vi "Begin.vi"(8 "error in":errorcluster) -> (0 "error out":errorcluster)   [LabVIEW 2020]
doc: "Called before other user functions, this VI is expected to open initial I/O refnums, load in file data, and do all program initialization. Notice that the <B>error out</B> terminal is simply used for data flow. Wiring it to other structures or subVIs ensures that this VI runs first."
uses:
  <vilib>/Rock Robotics/WPI/ThirdParty/Phoenix-LabVIEW/CANCoder/Controls/CTRE_Phoenix_CANcoder_Configurables.ctl
  <vilib>/Rock Robotics/WPI/ThirdParty/Phoenix-LabVIEW/CANCoder/Controls/CTRE_Phoenix_CANcoder_SensorInitializationStrategy.ctl
  <vilib>/Rock Robotics/WPI/ThirdParty/Phoenix-LabVIEW/CANCoder/Controls/CTRE_Phoenix_CANcoder_AbsoluteSensorRange.ctl
  <vilib>/Rock Robotics/WPI/ThirdParty/Phoenix-LabVIEW/Motor Controller/Controls/CTRE_Phoenix_MotorControl_VelocityMeasurementPeriod.ctl
  <vilib>/Rock Robotics/WPI/ThirdParty/Phoenix-LabVIEW/CANCoder/Controls/CTRE_Phoenix_CANcoder_SensorTimeBase.ctl
  <vilib>/Rock Robotics/WPI/DriverStation/WPI_DriverStationRobotMode2.ctl
  <vilib>/Rock Robotics/WPI/Joystick/WPI_JoystickDeviceEnum.ctl
  <vilib>/Rock Robotics/WPI/ThirdParty/Phoenix-LabVIEW/Pigeon IMU/CTRE_PigeonIMU_TareType.ctl
  <vilib>/Rock Robotics/WPI/ThirdParty/Phoenix-LabVIEW/Motor Controller/Controls/CTRE_Phoenix_MotorControl_TalonFXInvertType.ctl
  <vilib>/Rock Robotics/WPI/ThirdParty/Phoenix-LabVIEW/Motor Controller/Controls/CTRE_Phoenix_MotorControl_NeutralMode.ctl
  <vilib>/Rock Robotics/WPI/ThirdParty/Phoenix-LabVIEW/Motor Controller/Controls/CTRE_Phoenix_MotorControl_SupplyCurrentLimitConfiguration.ctl
  <vilib>/Rock Robotics/WPI/ThirdParty/Phoenix-LabVIEW/Motor Controller/Controls/CTRE_Phoenix_MotorControl_FeedbackDevice_TalonFX.ctl
  <vilib>/Rock Robotics/WPI/ThirdParty/REV Robotics/REVLib/Typedef/Spark MAX Idle Mode.ctl
  <vilib>/Rock Robotics/WPI/ThirdParty/REV Robotics/REVLib/Typedef/Spark MAX Limit Direction.ctl
  <vilib>/Rock Robotics/WPI/ThirdParty/Phoenix-LabVIEW/Motor Controller/Controls/CTRE_Phoenix_MotorControl_FeedbackDevice.ctl
  <vilib>/Rock Robotics/SystemInterfaces/DIO/FPGA_DIOChannel.ctl
  <vilib>/Rock Robotics/SystemInterfaces/AnalogTrigger/FPGA_AnalogTriggerOutType.ctl
  <vilib>/Rock Robotics/SystemInterfaces/DIO/FPGA_DIOPWMChannel.ctl
  <vilib>/Rock Robotics/WPI/ThirdParty/JAS_Junk/TrajLib/Rotation2d_CreateAngle.vi
  <vilib>/Rock Robotics/WPI/ThirdParty/JAS_Junk/TrajLib/Translation2d_Create.vi
  Robot Global Data.vi
  <vilib>/Rock Robotics/WPI/ThirdParty/Phoenix-LabVIEW/CANCoder/Set/CTRE_Phoenix_CANcoder_SetPositionToAbsolute.vi
  <vilib>/Rock Robotics/WPI/Counter/WPI_CounterDigitalInputToDigitalSource.vi
  <vilib>/Rock Robotics/WPI/AnalogTrigger/WPI_AnalogTriggerOpen_DutyCycle.vi
  <vilib>/Rock Robotics/WPI/Counter/WPI_CounterAnalogTriggerToDigitalSource.vi
  <vilib>/Rock Robotics/WPI/Counter/WPI_CounterOpen UpDown Mode.vi
  <vilib>/Rock Robotics/WPI/MotorControl/WPI_MotorControlOpen SPARK.vi
  <vilib>/Rock Robotics/WPI/ThirdParty/JAS_Junk/TrajLib/Trajectory_Library.lvlib
panel:
  in  "CANcoder ID1":T1={"Sensor Initialization Strategy"=enum."Boot To Absolute Position", "Absolute Sensor Range"=enum."Signed [-180 to +180)", "Velocity Measurement Period"=100, "Velocity Measurement Window"=64, "Magnet Offset (Degrees)"=85.0, "Sensor Direction"=FALSE, "Sensor Coefficient"=0.087890625, "Unit String"="deg", "Sensor Time Base"=enum."PerMinute"} {"Velocity Measurement Period" items=["Period_1ms"=1, "Period_2ms"=2, "Period_5ms"=5, "Period_10ms"=10, "Period_20ms"=20, "Period_25ms"=25, "Period_50ms"=50, "Period_100ms"=100]; "Sensor Coefficient" format="%#_9g"}
  in  "CANcoder ID0":T1={"Sensor Initialization Strategy"=enum."Boot To Absolute Position", "Absolute Sensor Range"=enum."Signed [-180 to +180)", "Velocity Measurement Period"=100, "Velocity Measurement Window"=64, "Magnet Offset (Degrees)"=116.0, "Sensor Direction"=FALSE, "Sensor Coefficient"=0.087890625, "Unit String"="deg", "Sensor Time Base"=enum."PerMinute"} {"Velocity Measurement Period" items=["Period_1ms"=1, "Period_2ms"=2, "Period_5ms"=5, "Period_10ms"=10, "Period_20ms"=20, "Period_25ms"=25, "Period_50ms"=50, "Period_100ms"=100]; "Sensor Coefficient" format="%#_9g"}
  in  "CANcoder ID2":T1={"Sensor Initialization Strategy"=enum."Boot To Absolute Position", "Absolute Sensor Range"=enum."Signed [-180 to +180)", "Velocity Measurement Period"=100, "Velocity Measurement Window"=64, "Magnet Offset (Degrees)"=-75.0, "Sensor Direction"=FALSE, "Sensor Coefficient"=0.087890625, "Unit String"="deg", "Sensor Time Base"=enum."PerMinute"} {"Velocity Measurement Period" items=["Period_1ms"=1, "Period_2ms"=2, "Period_5ms"=5, "Period_10ms"=10, "Period_20ms"=20, "Period_25ms"=25, "Period_50ms"=50, "Period_100ms"=100]; "Sensor Coefficient" format="%#_9g"}
  in  "CANcoder ID3":T1={"Sensor Initialization Strategy"=enum."Boot To Absolute Position", "Absolute Sensor Range"=enum."Signed [-180 to +180)", "Velocity Measurement Period"=100, "Velocity Measurement Window"=-116, "Magnet Offset (Degrees)"=-134.0, "Sensor Direction"=FALSE, "Sensor Coefficient"=0.087890625, "Unit String"="deg", "Sensor Time Base"=enum."PerMinute"} {"Velocity Measurement Period" items=["Period_1ms"=1, "Period_2ms"=2, "Period_5ms"=5, "Period_10ms"=10, "Period_20ms"=20, "Period_25ms"=25, "Period_50ms"=50, "Period_100ms"=100]; "Sensor Coefficient" format="%#_9g"}
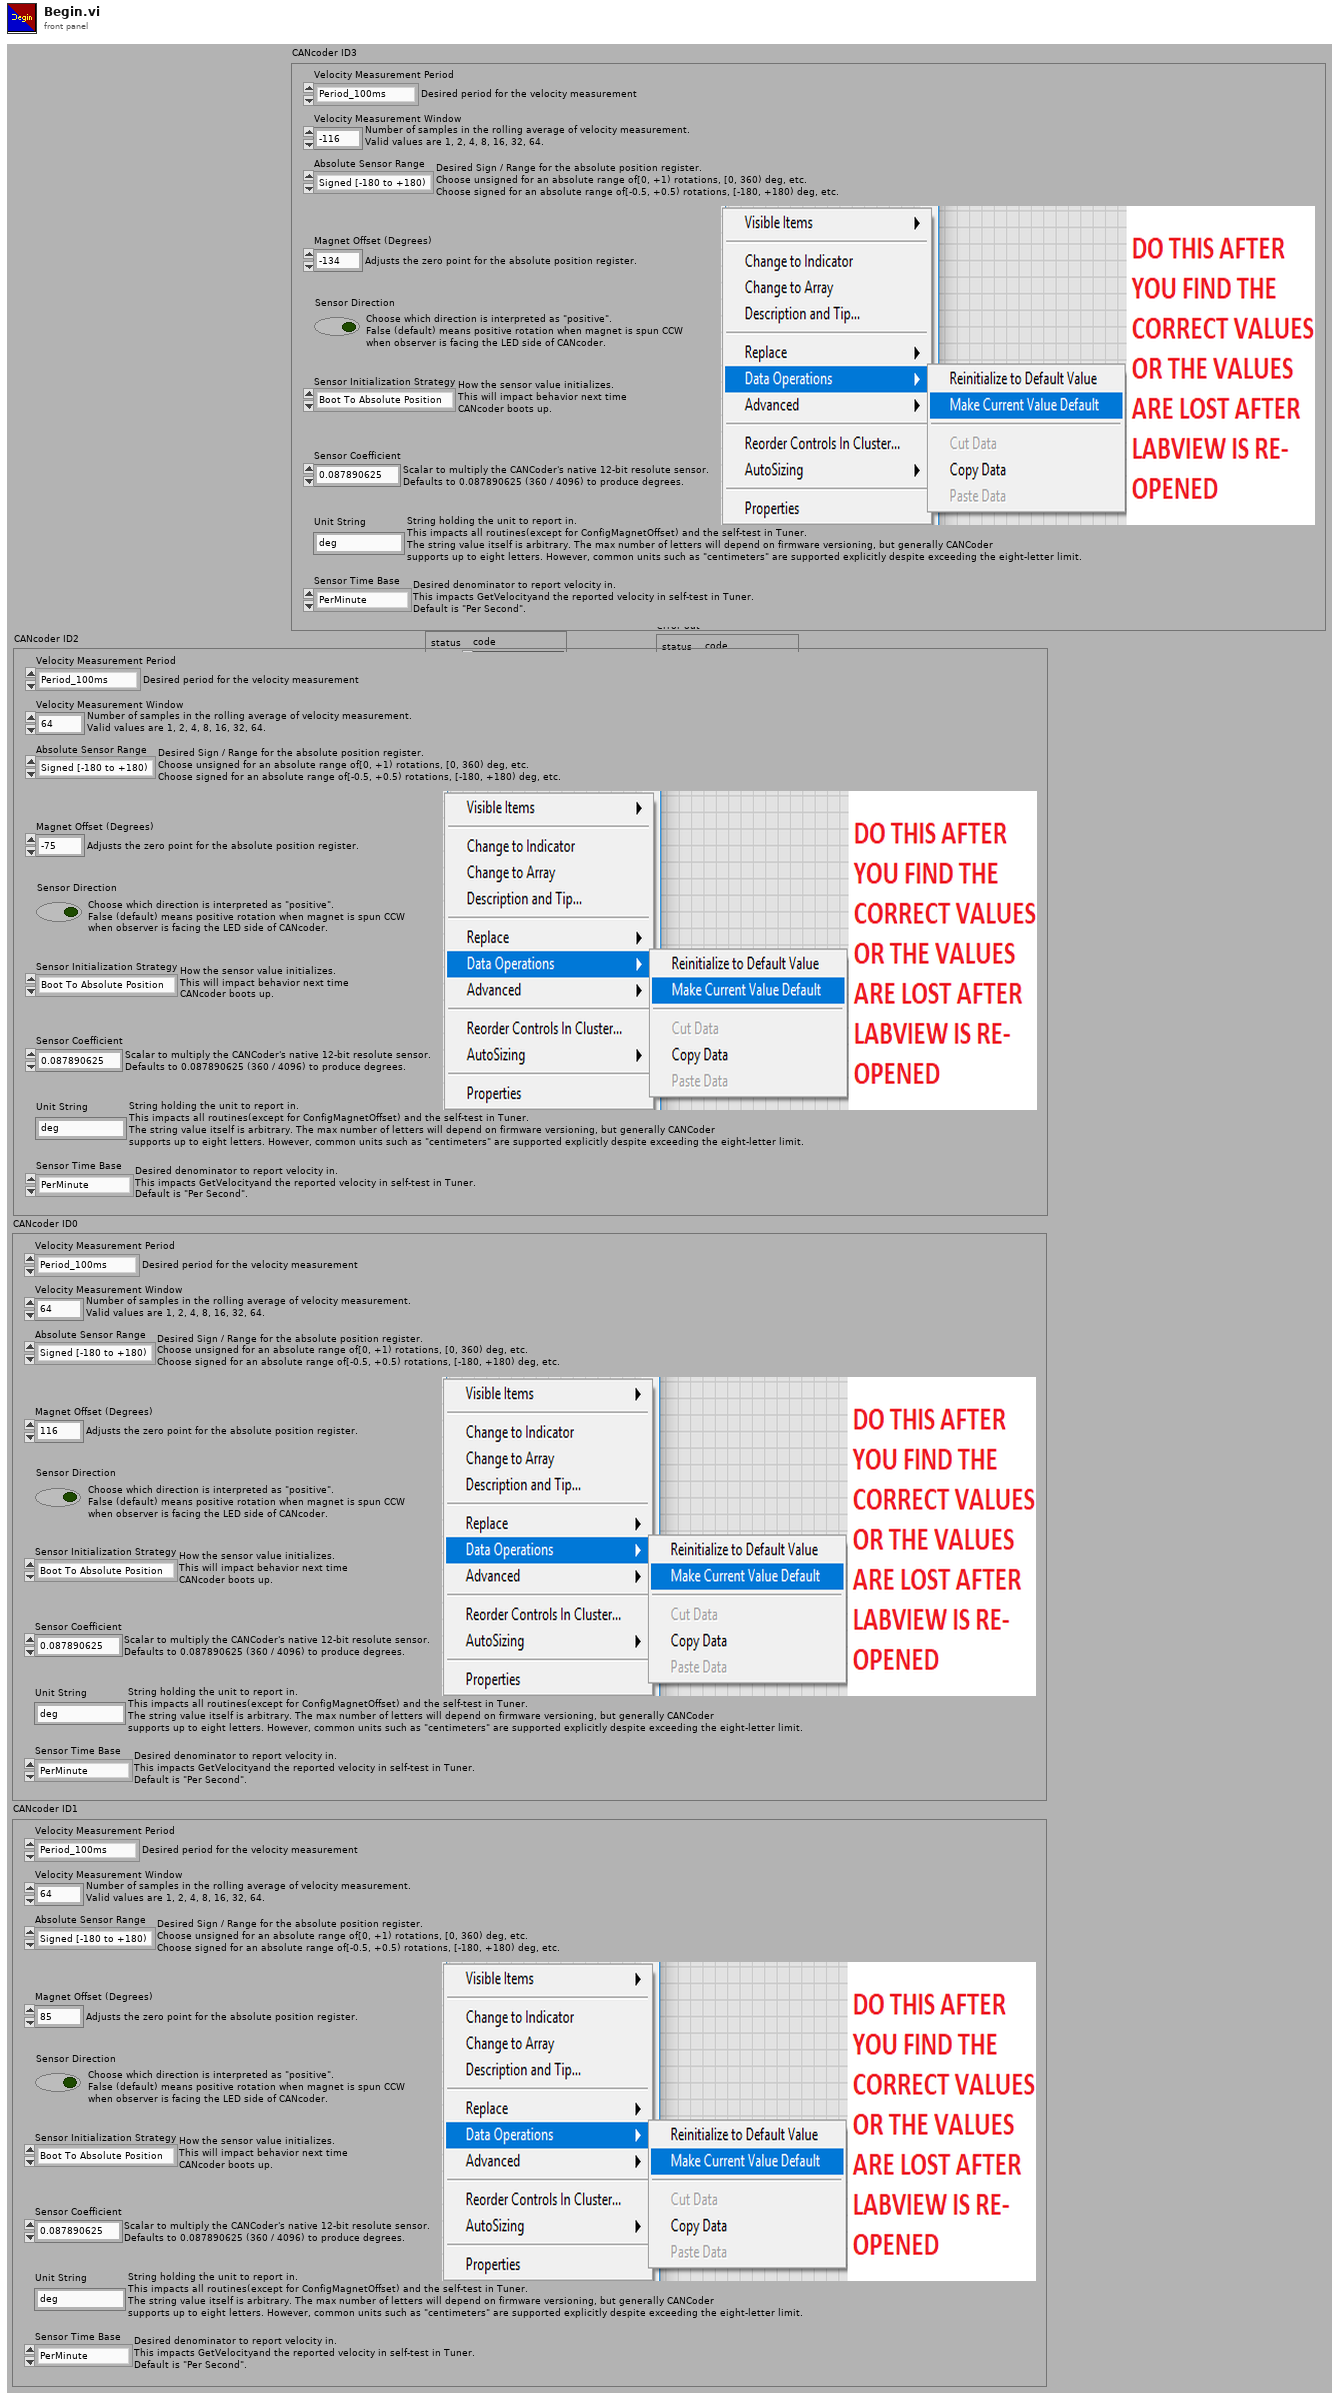
[diagram p1: front panel]
types:
  T1 = typedef "CTRE_Phoenix_CANcoder_Configurables.ctl" = cluster{"Sensor Initialization Strategy":T2, "Absolute Sensor Range":T3, "Velocity Measurement Period":T4, "Velocity Measurement Window":i32, "Magnet Offset (Degrees)":dbl, "Sensor Direction":bool, "Sensor Coefficient":dbl, "Unit String":string, "Sensor Time Base":T5}
  T2 = typedef "CTRE_Phoenix_CANcoder_SensorInitializationStrategy.ctl" = enum16{"Boot To Zero", "Boot To Absolute Position"}
  T3 = typedef "CTRE_Phoenix_CANcoder_AbsoluteSensorRange.ctl" = enum16{"Unsigned [0 to 360)", "Signed [-180 to +180)"}
  T4 = typedef "CTRE_Phoenix_MotorControl_VelocityMeasurementPeriod.ctl" = u16
  T5 = typedef "CTRE_Phoenix_CANcoder_SensorTimeBase.ctl" = enum16{"Per100Ms_Legacy", "PerSecond", "PerMinute"}
  T6 = typedef "FPGA_DIOPWMChannel.ctl" = enum8{"PWM 0", "PWM 1", "PWM 2", "PWM 3", "PWM 4", "PWM 5", "PWM 6", "PWM 7", "PWM 8", "PWM 9", "PWM MXP 0", "PWM MXP 1", "PWM MXP 2", "PWM MXP 3", "PWM MXP 4", "PWM MXP 5", "PWM MXP 6", "PWM MXP 7", "PWM MXP 8", "PWM MXP 9", "Invalid"}
  T7 = enum16{"Rising Edge", "Falling Edge", "Raising & Falling Edge", "Disabled"}
  T8 = typedef "FPGA_AnalogTriggerOutType.ctl" = enum16{"InWindow", "TriggerState", "Rising", "Falling"}
  T9 = typedef "FPGA_DIOChannel.ctl" = enum8{"DIO 0", "DIO 1", "DIO 2", "DIO 3", "DIO 4", "DIO 5", "DIO 6", "DIO 7", "DIO 8", "DIO 9", "DIO MXP 0", "DIO MXP 1", "DIO MXP 2", "DIO MXP 3", "DIO MXP 4", "DIO MXP 5", "DIO MXP 6", "DIO MXP 7", "DIO MXP 8", "DIO MXP 9", "DIO MXP 10", "DIO MXP 11", "DIO MXP 12", "DIO MXP 13", "DIO MXP 14", "DIO MXP 15", "SPI Port CS1", "SPI Port CS2", "SPI Port CS3", "SPI Port MISO", "SPI Port MOSI", "Invalid"}
  T10 = typedef "CTRE_Phoenix_MotorControl_FeedbackDevice.ctl" = i8
  T11 = typedef "CTRE_Phoenix_MotorControl_NeutralMode.ctl" = enum8{"EEPROMSetting", "Override to Coast", "Override to Brake"}
  T12 = typedef "Spark MAX Limit Direction.ctl" = enum16{"Forward Limit", "Reverse Limit"}
  T13 = typedef "Spark MAX Idle Mode.ctl" = enum16{"Coast", "Brake"}
  T14 = typedef "CTRE_Phoenix_MotorControl_TalonFXInvertType.ctl" = enum16{"Counter-Clockwise", "Clockwise"}
  T15 = typedef "CTRE_Phoenix_MotorControl_FeedbackDevice_TalonFX.ctl" = i8
  T16 = typedef "CTRE_Phoenix_MotorControl_SupplyCurrentLimitConfiguration.ctl" = cluster{"Enable?":bool, "Current Limit":dbl, "Threshold Current":dbl, "Threshold Time":dbl}
  T17 = typedef "CTRE_PigeonIMU_TareType.ctl" = u8
  T18 = typedef "WPI_JoystickDeviceEnum.ctl" = enum16{"USB 0", "USB 1", "USB 2", "USB 3", "USB 4", "USB 5"}
  T19 = typedef "WPI_DriverStationRobotMode2.ctl" = enum16{"Autonomous Disabled", "Autonomous Enabled", "Teleop Disabled", "Teleop Enabled", "Disconnected", "Finish", "Test Disabled", "Test Enabled", "Emergency Stopped"}
  T20 = typedef "Trajectory_Library.lvlib/ROTATION2D.ctl" = cluster{"VALUE":dbl, "COS":dbl, "SIN":dbl}
  T21 = typedef "Trajectory_Library.lvlib/SWERVE_DRIVE_MODULE_POSITION.ctl" = cluster{"Distance":dbl, "Angle":T20, "P":bool}
  T22 = typedef "Trajectory_Library.lvlib/POSE2D.ctl" = cluster{"TRANSLATION":T23, "ROTATION":T20}
  T23 = typedef "Trajectory_Library.lvlib/TRANSLATION2D.ctl" = cluster{"X":dbl, "Y":dbl}
  T24 = typedef "WPI_JoystickDevRef.ctl" = cluster{"Device":T18}
  T25 = typedef "Trajectory_Library.lvlib/SWERVE_DRIVE_ODOMETRY.ctl" = cluster{"POSE":T22, "GyroOffset":T20, "PreviousAngle":T20, "PrevModulePositions":T21[], "NumModules":i32}
  T26 = typedef "WPI_DigitalInputDevRef.ctl" = cluster{"DevStatus":errorcluster, "DIO Channel":T9}
  T27 = typedef "FPGA_CounterEncoderSourceConvertionLVSourceType.ctl" = cluster{"DevStatus":errorcluster, "AnalogTriggerMode?":bool, "DigitalMode":cluster{"DIO Channel":T28}, "AnalogTriggerMode":cluster{"AnalogTriggerIndex":T29, "OutputType":T8}}
  T28 = typedef "FPGA_DIODigitalSourceChannel.ctl" = enum8{"DIO 0", "DIO 1", "DIO 2", "DIO 3", "DIO 4", "DIO 5", "DIO 6", "DIO 7", "DIO 8", "DIO 9", "DIO MXP 0", "DIO MXP 1", "DIO MXP 2", "DIO MXP 3", "DIO MXP 4", "DIO MXP 5", "DIO MXP 6", "DIO MXP 7", "DIO MXP 8", "DIO MXP 9", "DIO MXP 10", "DIO MXP 11", "DIO MXP 12", "DIO MXP 13", "DIO MXP 14", "DIO MXP 15", "SPI Port CS1", "SPI Port CS2", "SPI Port CS3", "SPI Port MISO", "SPI Port MOSI", "Disabled"}
  T29 = typedef "FPGA_AnalogTriggerIndex.ctl" = enum8{"Trig 0", "Trig 1", "Trig 2", "Trig 3", "Trig 4", "Trig 5", "Trig 6", "Trig 7", "Invalid"}
  T30 = typedef "FPGA_DutyCycleDevRef.ctl" = cluster{"DevStatus":errorcluster, "DutyCycleIndex":T31}
  T31 = typedef "FPGA_DutyCycleIndex.ctl" = enum8{"DutyCycle 0", "DutyCycle 1", "DutyCycle 2", "DutyCycle 3", "DutyCycle 4", "DutyCycle 5", "DutyCycle 6", "DutyCycle 7", "Invalid"}
  T32 = typedef "WPI_MotorControlDeviceRef.ctl" = cluster{"DeviceStatus":errorcluster, "Type":T33, "PWM":cluster{"PWM Channel":T6, "DeadBand":T34}, "CAN":cluster{"Device Number":u8, "SetOutput VI Ref":variant, "GetOutput VI Ref":variant, "Enable VI Ref":variant, "Disable VI Ref":variant, "Data":variant}, "Invert":bool, "DIO PWM":cluster{"PWM \"Enable\" Channel":T6, "DIOChannel":T9, "PWM Rate":dbl}}
  T33 = typedef "WPI_MotorControlType.ctl" = enum16{"PWM", "CAN", "DIO PWM"}
  T34 = typedef "WPI_PWMDeadband.ctl" = cluster{"Name":string, "maxPositivePwm":i32, "minPositivePwm":i32, "centerPwm":i32, "maxNegativePwm":i32, "minNegativePwm":i32, "angularRange":u16}
  T35 = typedef "FPGA_AnalogTriggerDevRef.ctl" = cluster{"DevStatus":errorcluster, "AnalogTriggerIndex":T29}
  T36 = typedef "CTRE_PigeonIMU_DeviceRef.ctl" = cluster{"DeviceStatus":errorcluster, "Device Number":u8, "Type":T37, "Device ID":u32, "Handle":u64, "UsageFrame":u32, "Library Path":path}
  T37 = typedef "CTRE_PigeonIMU_ConnectionType.ctl" = u32
  T38 = typedef "CTRE_Phoenix_CANcoder_DeviceRef.ctl" = cluster{"DeviceStatus":errorcluster, "Device Number":u8, "Handle":u64, "UsageFrame":u32, "Library Path":path}
  T39 = typedef "WPI_CounterDevRef.ctl" = cluster{"DevStatus":errorcluster, "CntIndex":T40}
  T40 = typedef "FPGA_CounterCtrSystemIndex.ctl" = enum8{"Ctr 0", "Ctr 1", "Ctr 2", "Ctr 3", "Ctr 4", "Ctr 5", "Ctr 6", "Ctr 7", "Invalid"}
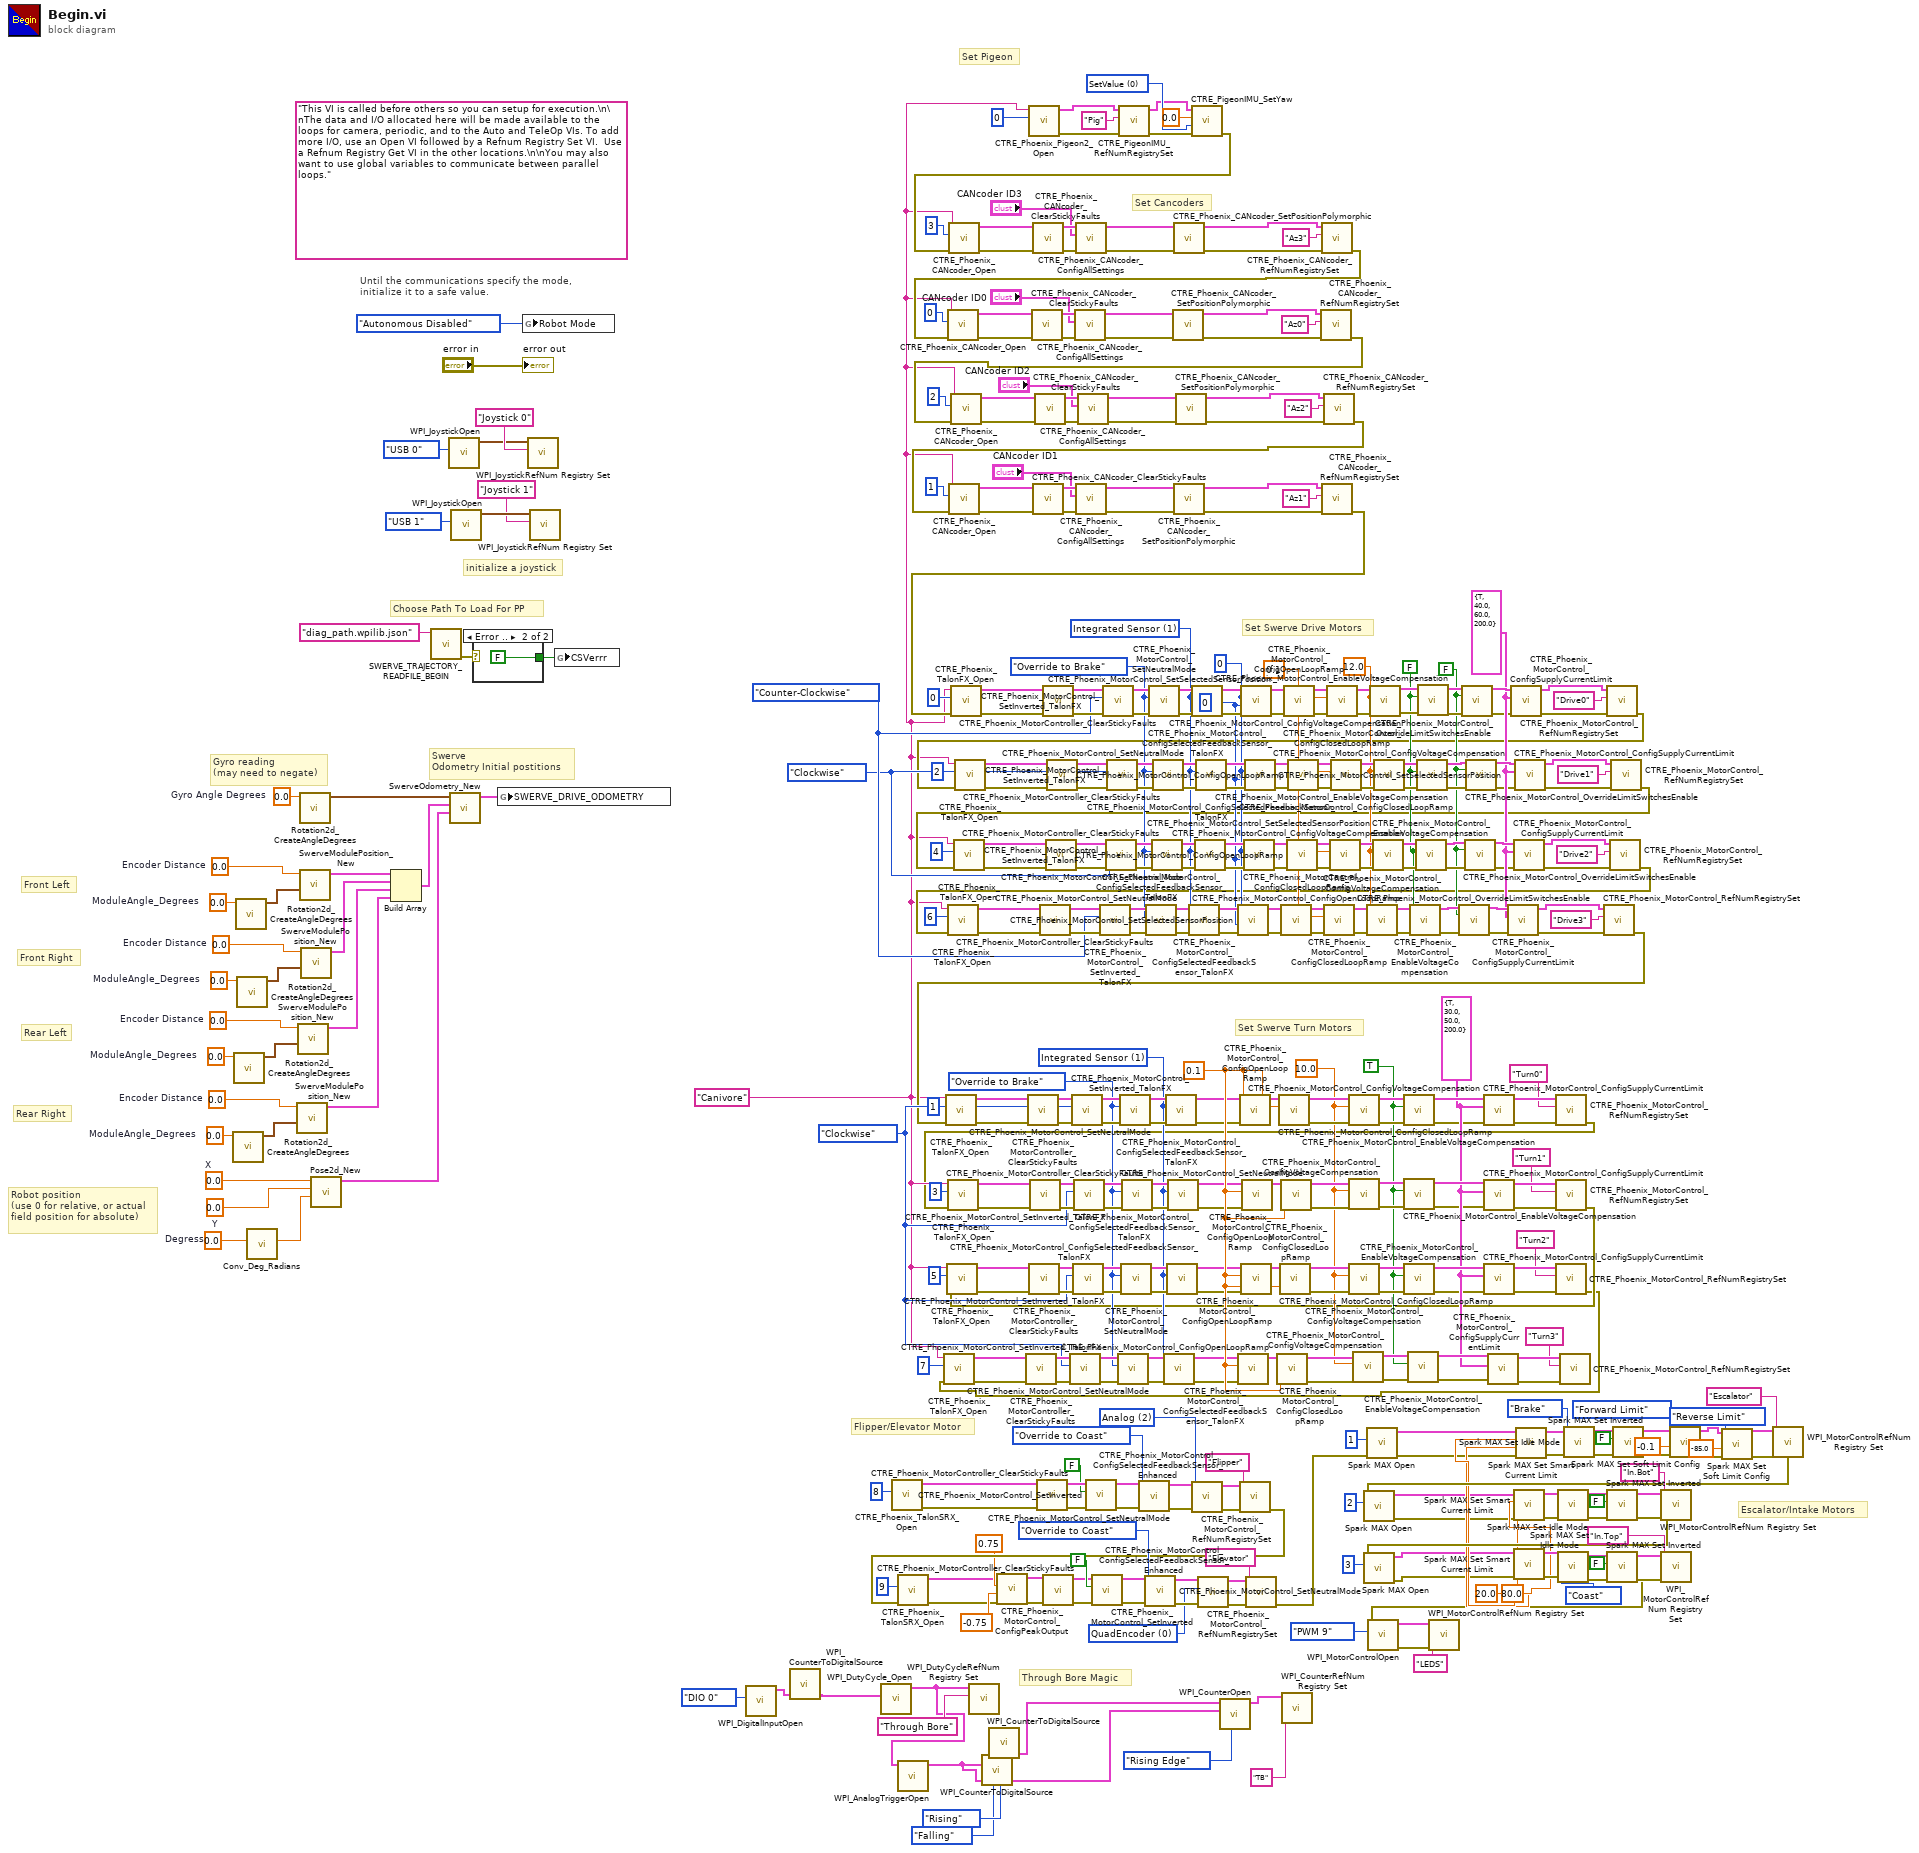
[diagram p0: block diagram]
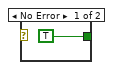
[diagram p2: hidden frame]
diagram:
  w42 = 20.0 ("Free Speed Current Limit (20A)")
  w43 = 80.0 ("Primay Current Limit (80A)")
  w67 = T10 0 items=["QuadEncoder"=0, "Analog"=2, "Tachometer"=4, "Pulse Width Encoded Position"=8, "Sensor Sum (S0 + S1)"=9, "Sensor Difference (D0 - D1)"=10, "Remote Source 0"=11, "Remote Source 1"=12, "Software Emulated"=15] ("Feedback Device")
  w81 = T10 2 items=["QuadEncoder"=0, "Analog"=2, "Tachometer"=4, "Pulse Width Encoded Position"=8, "Sensor Sum (S0 + S1)"=9, "Sensor Difference (D0 - D1)"=10, "Remote Source 0"=11, "Remote Source 1"=12, "Software Emulated"=15] ("Feedback Device")
  w123 = "Canivore" ("CAN Bus")
  w153 = 0.0  # Degress
  w152 = 0.0  # X
  w151 = 0.0  # Y
  w148 = 0.0  # ModuleAngle_Degrees
  w146 = 0.0  # Encoder Distance
  w145 = 0.0  # ModuleAngle_Degrees
  w143 = 0.0  # Encoder Distance
  w142 = 0.0  # ModuleAngle_Degrees
  w140 = 0.0  # Encoder Distance
  w139 = 0.0  # Gyro Angle Degrees
  w138 = 0.0  # ModuleAngle_Degrees
  w136 = 0.0  # Encoder Distance
  w159 = CTRE_Phoenix_MotorControl_TalonFXInvertType."Clockwise" ("Invert Type")
  w194 = TRUE ("Enable Voltage Compensation?")
  w195 = 10.0 ("Saturation Voltage")
  w193 = T15 1 items=["Integrated Sensor"=1, "Sensor Sum (S0 + S1)"=9, "Sensor Difference (D0 - D1)"=10, "Remote Source 0"=11, "Remote Source 1"=12, "None"=14, "Software Emulated"=15] ("Talon FX Feedback Device")
  w180 = T16 {"Enable?"=TRUE, "Current Limit"=30.0, "Threshold Current"=50.0, "Threshold Time"=200.0} ("Supply Current Limit Configuration")
  w212 = 0.1 ("secondsFromNeutralToFull")
  w213 = CTRE_Phoenix_MotorControl_NeutralMode."Override to Brake" ("Motor Control Neutral Mode")
  w270 = FALSE ("Override Limit Switch Enable?")
  w247 = CTRE_Phoenix_MotorControl_TalonFXInvertType."Counter-Clockwise" ("Invert Type")
  w279 = FALSE ("Enable Voltage Compensation?")
  w280 = 12.0 ("Saturation Voltage")
  w269 = T15 1 items=["Integrated Sensor"=1, "Sensor Sum (S0 + S1)"=9, "Sensor Difference (D0 - D1)"=10, "Remote Source 0"=11, "Remote Source 1"=12, "None"=14, "Software Emulated"=15] ("Talon FX Feedback Device")
  w256 = T16 {"Enable?"=TRUE, "Current Limit"=40.0, "Threshold Current"=60.0, "Threshold Time"=200.0} ("Supply Current Limit Configuration")
  w297 = 0.1 ("secondsFromNeutralToFull")
  w298 = u32 0 ("pidLoopIdx")
  w299 = 0 ("New Sensor Position")
  w300 = CTRE_Phoenix_MotorControl_NeutralMode."Override to Brake" ("Motor Control Neutral Mode")
  w246 = CTRE_Phoenix_MotorControl_TalonFXInvertType."Clockwise" ("Invert Type")
  w397 = T17 0 items=["SetValue"=0, "AddOffset"=1, "MatchCompass"=2, "SetOffset"=255] ("TareType (SetValue)")
  (unwired) "This VI is called before others so you can setup for execution.\n\nThe data and I/O allocated here will be made available to the loops for camera, periodic, and to the Auto and TeleOp VIs. To add more I/O, use an Open VI followed by a Refnum Registry Set VI.  Use a Refnum Registry Get VI in the other locations.\n\nYou may also want to use global variables to communicate between parallel loops."
  # "Choose Path To Load For PP"
  # "Through Bore Magic"
  # "Escalator/Intake Motors"
  # "Flipper/Elevator Motor"
  # "Set Swerve Turn Motors"
  # "Set Swerve Drive Motors"
  # "Set Cancoders"
  # "Set Pigeon"
  # "Swerve\nOdometry Initial postitions"
  # "Robot position\n(use 0 for relative, or actual \nfield position for absolute)"
  # "Rear Right"
  # "Rear Left"
  # "Front Right"
  # "Front Left"
  # "Gyro reading\n(may need to negate)"
  # "initialize a joystick"
  # "Until the communications specify the mode,\ninitialize it to a safe value."
  n1 = call <vilib>:"Rotation2d_CreateAngleDegrees.vi"("Angle_Degrees"=w148) -> ("ROTATION"=w147:T20)  [unwired: 10 in]
  n2 = call <vilib>:"Rotation2d_CreateAngleDegrees.vi"("Angle_Degrees"=w145) -> ("ROTATION"=w144:T20)  [unwired: 10 in]
  n3 = call <vilib>:"Rotation2d_CreateAngleDegrees.vi"("Angle_Degrees"=w138) -> ("ROTATION"=w137:T20)  [unwired: 10 in]
  n4 = call <vilib>:"Rotation2d_CreateAngleDegrees.vi"("Angle_Degrees"=w142) -> ("ROTATION"=w141:T20)  [unwired: 10 in]
  n5 = call <vilib>:"Conv_Deg_Radians.vi"("Degress"=w153) -> ("Radians"=w150:dbl)  [unwired: 10 in]
  n6 = call <vilib>:"SwerveModulePosition_New.vi"("ROTATION"=w147, "Distance"=w146) -> ("SWERVE_DRIVE_MODULE_POSITION"=w131:T21)  [unwired: 9 in]
  n7 = call <vilib>:"SwerveModulePosition_New.vi"("ROTATION"=w144, "Distance"=w143) -> ("SWERVE_DRIVE_MODULE_POSITION"=w132:T21)  [unwired: 9 in]
  n8 = call <vilib>:"Rotation2d_CreateAngleDegrees.vi"("Angle_Degrees"=w139) -> ("ROTATION"=w149:T20)  [unwired: 10 in]
  n9 = call <vilib>:"SwerveModulePosition_New.vi"("ROTATION"=w137, "Distance"=w136) -> ("SWERVE_DRIVE_MODULE_POSITION"=w134:T21)  [unwired: 9 in]
  n10 = call <vilib>:"SwerveModulePosition_New.vi"("ROTATION"=w141, "Distance"=w140) -> ("SWERVE_DRIVE_MODULE_POSITION"=w133:T21)  [unwired: 9 in]
  n11 = call <vilib>:"Pose2d_New.vi"("Heading"=w150, "Y"=w151, "X"=w152) -> ("out POSe"=w154:T22)  [unwired: 8 in]
  n12 = Build Array(w134, w133, w132, w131) -> (w130:T21[])
  n13 = call "SWERVE_TRAJECTORY_READFILE_BEGIN.vi"("Trajectory File Name"="diag_path.wpilib.json") -> ("error out"=w157:errorcluster)  [unwired: 8 in, 2 out]
  n14 = call <vilib>:"WPI_JoystickOpen.vi"("JoystickDevice"=WPI_JoystickDeviceEnum."USB 0") -> ("JoystickDevRef"=w406:T24)  [unwired: 10 in]
  n15 = call <vilib>:"SwerveOdometry_New.vi"("InitialPose"=w154, "Module Positions"=w130, "gyroAngle"=w149) -> ("SWERVE_DRIVE_ODOMETRY"=w135:T25)  [unwired: 8 in]
  n16 = call <vilib>:"WPI_JoystickOpen.vi"("JoystickDevice"=WPI_JoystickDeviceEnum."USB 1") -> ("JoystickDevRef"=w402:T24)  [unwired: 10 in]
  n17 = case shown="Error .." w157 {
    tunnel: [TRUE FALSE] -> w156
    frame No Error {
    }
    frame Error {
    }
  }
  n18 = global write "Robot Global Data.vi" "SWERVE_DRIVE_ODOMETRY"(w135) -> ()
  n19 = global write "Robot Global Data.vi" "Robot Mode"(WPI_DriverStationRobotMode2."Autonomous Disabled" ("Robot Mode")) -> ()
  n20 = call <vilib>:"WPI_JoystickRefNum Registry Set.vi"("refnum name"="Joystick 0", "JoystickDevRef"=w406) -> ()  [unwired: 8 in, 2 out]
  n21 = call <vilib>:"WPI_JoystickRefNum Registry Set.vi"("refnum name"="Joystick 1", "JoystickDevRef"=w402) -> ()  [unwired: 8 in, 2 out]
  n22 = global write "Robot Global Data.vi" "CSVerrr"(w156) -> ()
  n23 = call <vilib>:"WPI_DigitalInputOpen.vi"("DIO Channel"=FPGA_DIOChannel."DIO 0") -> ("DigitalInputDevRef"=w64:T26)  [unwired: 9 in, 1 out]
  n24 = call-poly <vilib>:"WPI_CounterToDigitalSource.vi"("DigitalInputDevRef"=w64) -> ("Digital Source"=w63:T27)  [unwired: 6 in]
  n25 = call <vilib>:"WPI_DutyCycle_Open.vi"("Source"=w63) -> ("DutyCycleDevRef"=w61:T30)  [unwired: 9 in, 1 out]
  n26 = call <vilib>:"CTRE_Phoenix_TalonSRX_Open.vi"("Device Number"=u8 8) -> ("error out"=w94:errorcluster, "PhoenixMotorControlDevRef"=w93:T32)  [unwired: 9 in]
  n27 = call-poly <vilib>:"WPI_AnalogTriggerOpen.vi"("AnalogTriggerSource"=w61) -> ("AnalogTriggerDevRef"=w60:T35)  [unwired: 9 in, 1 out]
  n28 = call <vilib>:"WPI_DutyCycleRefNum Registry Set.vi"("refnum name"="Through Bore", "DutyCycleDevRef"=w61) -> ()  [unwired: 8 in, 2 out]
  n29 = call-poly <vilib>:"WPI_CounterToDigitalSource.vi"("AnalogTriggerDevRef"=w60, "OutputType"=FPGA_AnalogTriggerOutType."Falling") -> ("Digital Source"=w56:T27)  [unwired: 5 in]
  n30 = call-poly <vilib>:"WPI_CounterToDigitalSource.vi"("AnalogTriggerDevRef"=w60, "OutputType"=FPGA_AnalogTriggerOutType."Rising") -> ("Digital Source"=w57:T27)  [unwired: 5 in]
  n31 = call <vilib>:"CTRE_Phoenix_Pigeon2_Open.vi"("Device Number"=u8 0, "canbus"=w123) -> ("error out"=w399:errorcluster, "PigeonIMUDevRef"=w400:T36)  [unwired: 8 in]
  n32 = call <vilib>:"CTRE_Phoenix_MotorController_ClearStickyFaults.vi"("error in"=w94, "PhoenixMotorControlDevRef"=w93) -> ("error out"=w92:errorcluster, "PhoenixMotorControlDevRef"=w91:T32)  [unwired: 8 in]
  n33 = call <vilib>:"CTRE_Phoenix_MotorControl_SetInverted.vi"("error in (no error)"=w92, "Invert?"=FALSE, "PhoenixMotorControlDevRef"=w91) -> ("error out"=w90:errorcluster, "PhoenixMotorControlDevRef"=w89:T32)  [unwired: 7 in]
  n34 = call <vilib>:"CTRE_PigeonIMU_RefNumRegistrySet.vi"("error in (no error)"=w399, "refnum name"="Pig", "PigeonIMUDevRef"=w400) -> ("error out"=w394:errorcluster, "PigeonIMUDevRef"=w395:T36)  [unwired: 7 in]
  n35 = call <vilib>:"CTRE_Phoenix_MotorControl_SetNeutralMode.vi"("error in (no error)"=w90, "Motor Control Neutral Mode"=CTRE_Phoenix_MotorControl_NeutralMode."Override to Coast", "PhoenixMotorControlDevRef"=w89) -> ("error out"=w88:errorcluster, "PhoenixMotorControlDevRef"=w87:T32)  [unwired: 7 in]
  n36 = call <vilib>:"CTRE_PigeonIMU_SetYaw.vi"("error in (no error)"=w394, "TareType (SetValue)"=w397, "Value"=0.0, "PigeonIMUDevRef"=w395) -> ("error out"=w356:errorcluster)  [unwired: 6 in, 1 out]
  n37 = call <vilib>:"CTRE_Phoenix_CANcoder_Open.vi"("error in"=w356, "Device Number"=u8 3, "CAN Bus"=w123) -> ("error out"=w7:errorcluster, "CTRE_CANcoder_DeviceRef"=w8:T38)  [unwired: 7 in]
  n38 = call <vilib>:"CTRE_Phoenix_CANcoder_ClearStickyFaults.vi"("error in"=w7, "CTRE_CANcoder_DeviceRef"=w8) -> ("error out"=w373:errorcluster, "CTRE_CANcoder_DeviceRef"=w374:T38)  [unwired: 8 in]
  n39 = call <vilib>:"CTRE_Phoenix_CANcoder_ConfigAllSettings.vi"("error in (no error)"=w373, "CANcoder Configurables"="CANcoder ID3", "CTRE_CANcoder_DeviceRef"=w374) -> ("error out"=w376:errorcluster, "CTRE_CANcoder_DeviceRef"=w375:T38)  [unwired: 7 in]
  n40 = call-poly <vilib>:"CTRE_Phoenix_CANcoder_SetPositionPolymorphic.vi"("error in (no error)"=w376, "CTRE_CANcoder_DeviceRef"=w375) -> ("error out"=w383:errorcluster, "CTRE_CANcoder_DeviceRef"=w384:T38)  [unwired: 8 in]
  n41 = call <vilib>:"CTRE_Phoenix_MotorControl_ConfigSelectedFeedbackSensor_Enhanced.vi"("error in (no error)"=w88, "Feedback Device"=w81, "PhoenixMotorControlDevRef"=w87) -> ("error out"=w86:errorcluster, "PhoenixMotorControlDevRef"=w85:T32)  [unwired: 7 in]
  n42 = call-poly <vilib>:"WPI_CounterOpen.vi"("DownEdge"=T7."Rising Edge", "Down Source"=w56, "Up Source"=w57) -> ("CounterDevRef"=w54:T39)  [unwired: 4 in, 4 out]
  n43 = call <vilib>:"CTRE_Phoenix_MotorControl_RefNumRegistrySet.vi"("error in (no error)"=w86, "refnum name"="Flipper", "PhoenixMotorControlDevRef"=w85) -> ("error out"=w68:errorcluster)  [unwired: 7 in, 1 out]
  n44 = call <vilib>:"CTRE_Phoenix_TalonSRX_Open.vi"("error in"=w68, "Device Number"=u8 9) -> ("error out"=w25:errorcluster, "PhoenixMotorControlDevRef"=w26:T32)  [unwired: 8 in]
  n45 = call <vilib>:"CTRE_Phoenix_MotorControl_ConfigPeakOutput.vi"("error in (no error)"=w25, "Reverse Peak Percent Output"=-0.75, "Forward Peak Percent Output"=0.75, "PhoenixMotorControlDevRef"=w26) -> ("error out"=w29:errorcluster, "PhoenixMotorControlDevRef"=w30:T32)  [unwired: 6 in]
  n46 = call <vilib>:"CTRE_Phoenix_MotorController_ClearStickyFaults.vi"("error in"=w29, "PhoenixMotorControlDevRef"=w30) -> ("error out"=w70:errorcluster, "PhoenixMotorControlDevRef"=w71:T32)  [unwired: 8 in]
  n47 = call <vilib>:"CTRE_Phoenix_MotorControl_SetInverted.vi"("error in (no error)"=w70, "Invert?"=FALSE, "PhoenixMotorControlDevRef"=w71) -> ("error out"=w72:errorcluster, "PhoenixMotorControlDevRef"=w73:T32)  [unwired: 7 in]
  n48 = call <vilib>:"CTRE_Phoenix_MotorControl_SetNeutralMode.vi"("error in (no error)"=w72, "Motor Control Neutral Mode"=CTRE_Phoenix_MotorControl_NeutralMode."Override to Coast", "PhoenixMotorControlDevRef"=w73) -> ("error out"=w74:errorcluster, "PhoenixMotorControlDevRef"=w75:T32)  [unwired: 7 in]
  n49 = call <vilib>:"CTRE_Phoenix_MotorControl_ConfigSelectedFeedbackSensor_Enhanced.vi"("error in (no error)"=w74, "Feedback Device"=w67, "PhoenixMotorControlDevRef"=w75) -> ("error out"=w76:errorcluster, "PhoenixMotorControlDevRef"=w77:T32)  [unwired: 7 in]
  n50 = call <vilib>:"CTRE_Phoenix_MotorControl_RefNumRegistrySet.vi"("error in (no error)"=w76, "refnum name"="Elevator", "PhoenixMotorControlDevRef"=w77) -> ("error out"=w66:errorcluster)  [unwired: 7 in, 1 out]
  n51 = call <vilib>:"WPI_CounterRefNum Registry Set.vi"("refnum name"="TB", "CounterDevRef"=w54) -> ()  [unwired: 8 in, 2 out]
  n52 = call <vilib>:"CTRE_Phoenix_CANcoder_RefNumRegistrySet.vi"("error in (no error)"=w383, "refnum name"="Az3", "CTRE_CANcoder_DeviceRef"=w384) -> ("error out"=w355:errorcluster)  [unwired: 7 in, 1 out]
  n53 = call <vilib>:"CTRE_Phoenix_CANcoder_Open.vi"("error in"=w355, "Device Number"=u8 0, "CAN Bus"=w123) -> ("error out"=w5:errorcluster, "CTRE_CANcoder_DeviceRef"=w6:T38)  [unwired: 7 in]
  n54 = call <vilib>:"CTRE_Phoenix_CANcoder_ClearStickyFaults.vi"("error in"=w5, "CTRE_CANcoder_DeviceRef"=w6) -> ("error out"=w364:errorcluster, "CTRE_CANcoder_DeviceRef"=w361:T38)  [unwired: 8 in]
  n55 = call <vilib>:"CTRE_Phoenix_CANcoder_ConfigAllSettings.vi"("error in (no error)"=w364, "CANcoder Configurables"="CANcoder ID0", "CTRE_CANcoder_DeviceRef"=w361) -> ("error out"=w363:errorcluster, "CTRE_CANcoder_DeviceRef"=w362:T38)  [unwired: 7 in]
  n56 = call-poly <vilib>:"CTRE_Phoenix_CANcoder_SetPositionPolymorphic.vi"("error in (no error)"=w363, "CTRE_CANcoder_DeviceRef"=w362) -> ("error out"=w381:errorcluster, "CTRE_CANcoder_DeviceRef"=w382:T38)  [unwired: 8 in]
  n57 = call <vilib>:"CTRE_Phoenix_CANcoder_RefNumRegistrySet.vi"("error in (no error)"=w381, "refnum name"="Az0", "CTRE_CANcoder_DeviceRef"=w382) -> ("error out"=w354:errorcluster)  [unwired: 7 in, 1 out]
  n58 = call <vilib>:"CTRE_Phoenix_CANcoder_Open.vi"("error in"=w354, "Device Number"=u8 2, "CAN Bus"=w123) -> ("error out"=w3:errorcluster, "CTRE_CANcoder_DeviceRef"=w4:T38)  [unwired: 7 in]
  n59 = call <vilib>:"CTRE_Phoenix_CANcoder_ClearStickyFaults.vi"("error in"=w3, "CTRE_CANcoder_DeviceRef"=w4) -> ("error out"=w365:errorcluster, "CTRE_CANcoder_DeviceRef"=w368:T38)  [unwired: 8 in]
  n60 = call <vilib>:"CTRE_Phoenix_CANcoder_ConfigAllSettings.vi"("error in (no error)"=w365, "CANcoder Configurables"="CANcoder ID2", "CTRE_CANcoder_DeviceRef"=w368) -> ("error out"=w366:errorcluster, "CTRE_CANcoder_DeviceRef"=w367:T38)  [unwired: 7 in]
  n61 = call-poly <vilib>:"CTRE_Phoenix_CANcoder_SetPositionPolymorphic.vi"("error in (no error)"=w366, "CTRE_CANcoder_DeviceRef"=w367) -> ("error out"=w380:errorcluster, "CTRE_CANcoder_DeviceRef"=w379:T38)  [unwired: 8 in]
  n62 = call <vilib>:"CTRE_Phoenix_CANcoder_RefNumRegistrySet.vi"("error in (no error)"=w380, "refnum name"="Az2", "CTRE_CANcoder_DeviceRef"=w379) -> ("error out"=w353:errorcluster)  [unwired: 7 in, 1 out]
  n63 = call <vilib>:"CTRE_Phoenix_CANcoder_Open.vi"("error in"=w353, "Device Number"=u8 1, "CAN Bus"=w123) -> ("error out"=w1:errorcluster, "CTRE_CANcoder_DeviceRef"=w2:T38)  [unwired: 7 in]
  n64 = call <vilib>:"CTRE_Phoenix_CANcoder_ClearStickyFaults.vi"("error in"=w1, "CTRE_CANcoder_DeviceRef"=w2) -> ("error out"=w372:errorcluster, "CTRE_CANcoder_DeviceRef"=w369:T38)  [unwired: 8 in]
  n65 = call <vilib>:"CTRE_Phoenix_CANcoder_ConfigAllSettings.vi"("error in (no error)"=w372, "CANcoder Configurables"="CANcoder ID1", "CTRE_CANcoder_DeviceRef"=w369) -> ("error out"=w371:errorcluster, "CTRE_CANcoder_DeviceRef"=w370:T38)  [unwired: 7 in]
  n66 = call-poly <vilib>:"CTRE_Phoenix_CANcoder_SetPositionPolymorphic.vi"("error in (no error)"=w371, "CTRE_CANcoder_DeviceRef"=w370) -> ("error out"=w377:errorcluster, "CTRE_CANcoder_DeviceRef"=w378:T38)  [unwired: 8 in]
  n67 = call <vilib>:"CTRE_Phoenix_CANcoder_RefNumRegistrySet.vi"("error in (no error)"=w377, "refnum name"="Az1", "CTRE_CANcoder_DeviceRef"=w378) -> ("error out"=w242:errorcluster)  [unwired: 7 in, 1 out]
  n68 = call <vilib>:"CTRE_Phoenix_TalonFX_Open.vi"("error in"=w242, "Device Number"=u8 0 ("Drive 4L"), "CAN Bus"=w123) -> ("error out"=w9:errorcluster, "PhoenixMotorControlDevRef"=w10:T32)  [unwired: 7 in]
  n69 = call <vilib>:"CTRE_Phoenix_MotorController_ClearStickyFaults.vi"("error in"=w9, "PhoenixMotorControlDevRef"=w10) -> ("error out"=w306:errorcluster, "PhoenixMotorControlDevRef"=w305:T32)  [unwired: 8 in]
  n70 = call <vilib>:"CTRE_Phoenix_MotorControl_SetInverted_TalonFX.vi"("error in (no error)"=w306, "Invert Type"=w247, "PhoenixMotorControlDevRef"=w305) -> ("error out"=w312:errorcluster, "PhoenixMotorControlDevRef"=w313:T32)  [unwired: 7 in]
  n71 = call <vilib>:"CTRE_Phoenix_MotorControl_SetNeutralMode.vi"("error in (no error)"=w312, "Motor Control Neutral Mode"=w300, "PhoenixMotorControlDevRef"=w313) -> ("error out"=w303:errorcluster, "PhoenixMotorControlDevRef"=w304:T32)  [unwired: 7 in]
  n72 = call <vilib>:"CTRE_Phoenix_MotorControl_ConfigSelectedFeedbackSensor_TalonFX.vi"("error in (no error)"=w303, "Talon FX Feedback Device"=w269, "PhoenixMotorControlDevRef"=w304) -> ("error out"=w301:errorcluster, "PhoenixMotorControlDevRef"=w302:T32)  [unwired: 7 in]
  n73 = call <vilib>:"CTRE_Phoenix_MotorControl_SetSelectedSensorPosition.vi"("error in (no error)"=w301, "pidLoopIdx"=w298, "New Sensor Position"=w299, "PhoenixMotorControlDevRef"=w302) -> ("error out"=w311:errorcluster, "PhoenixMotorControlDevRef"=w310:T32)  [unwired: 6 in]
  n74 = call <vilib>:"CTRE_Phoenix_MotorControl_ConfigOpenLoopRamp.vi"("error in (no error)"=w311, "secondsFromNeutralToFull"=w297, "PhoenixMotorControlDevRef"=w310) -> ("error out"=w307:errorcluster, "PhoenixMotorControlDevRef"=w308:T32)  [unwired: 7 in]
  n75 = call <vilib>:"CTRE_Phoenix_MotorControl_ConfigClosedLoopRamp.vi"("error in (no error)"=w307, "secondsFromNeutralToFull"=w297, "PhoenixMotorControlDevRef"=w308) -> ("error out"=w287:errorcluster, "PhoenixMotorControlDevRef"=w288:T32)  [unwired: 7 in]
  n76 = call <vilib>:"Spark MAX Open.vi"("error in (no error)"=w66, "Device Number"=u8 1) -> ("error out"=w37:errorcluster, "MotorControlDeviceRef"=w36:T32)  [unwired: 8 in]
  n77 = call <vilib>:"CTRE_Phoenix_MotorControl_ConfigVoltageCompensation.vi"("error in (no error)"=w287, "Saturation Voltage"=w280, "PhoenixMotorControlDevRef"=w288) -> ("error out"=w295:errorcluster, "PhoenixMotorControlDevRef"=w296:T32)  [unwired: 7 in]
  n78 = call <vilib>:"CTRE_Phoenix_MotorControl_EnableVoltageCompensation.vi"("error in (no error)"=w295, "Enable Voltage Compensation?"=w279, "PhoenixMotorControlDevRef"=w296) -> ("error out"=w277:errorcluster, "PhoenixMotorControlDevRef"=w278:T32)  [unwired: 7 in]
  n79 = call <vilib>:"CTRE_Phoenix_MotorControl_OverrideLimitSwitchesEnable.vi"("PhoenixMotorControlDevRef"=w278, "Override Limit Switch Enable?"=w270, "error in (no error)"=w277) -> ("PhoenixMotorControlDevRef"=w260:T32, "error out"=w251:errorcluster)  [unwired: 11 in]
  n80 = call <vilib>:"CTRE_Phoenix_MotorControl_ConfigSupplyCurrentLimit.vi"("error in (no error)"=w251, "Supply Current Limit Configuration"=w256, "PhoenixMotorControlDevRef"=w260) -> ("error out"=w261:errorcluster, "PhoenixMotorControlDevRef"=w262:T32)  [unwired: 7 in]
  n81 = call <vilib>:"Spark MAX Set Smart Current Limit.vi"("error in (no error)"=w37, "Free Speed Current Limit (20A)"=w42, "Primay Current Limit (80A)"=w43, "MotorControlDeviceRef in"=w36) -> ("error out"=w45:errorcluster, "MotorControlDeviceRef out"=w44:T32)  [unwired: 6 in]
  n82 = call <vilib>:"Spark MAX Set Idle Mode.vi"("error in (no error)"=w45, "Idle Mode"=Spark_MAX_Idle_Mode."Brake", "MotorControlDeviceRef in"=w44) -> ("error out"=w127:errorcluster, "MotorControlDeviceRef out"=w126:T32)  [unwired: 7 in]
  n83 = call <vilib>:"CTRE_Phoenix_MotorControl_RefNumRegistrySet.vi"("error in (no error)"=w261, "refnum name"="Drive0", "PhoenixMotorControlDevRef"=w262) -> ("error out"=w245:errorcluster)  [unwired: 7 in, 1 out]
  n84 = call <vilib>:"CTRE_Phoenix_TalonFX_Open.vi"("error in"=w245, "Device Number"=u8 2 ("Drive 4L"), "CAN Bus"=w123) -> ("error out"=w11:errorcluster, "PhoenixMotorControlDevRef"=w12:T32)  [unwired: 7 in]
  n85 = call <vilib>:"CTRE_Phoenix_MotorController_ClearStickyFaults.vi"("error in"=w11, "PhoenixMotorControlDevRef"=w12) -> ("error out"=w319:errorcluster, "PhoenixMotorControlDevRef"=w318:T32)  [unwired: 8 in]
  n86 = call <vilib>:"CTRE_Phoenix_MotorControl_SetInverted_TalonFX.vi"("error in (no error)"=w319, "Invert Type"=w246, "PhoenixMotorControlDevRef"=w318) -> ("error out"=w325:errorcluster, "PhoenixMotorControlDevRef"=w326:T32)  [unwired: 7 in]
  n87 = call <vilib>:"CTRE_Phoenix_MotorControl_SetNeutralMode.vi"("error in (no error)"=w325, "Motor Control Neutral Mode"=w300, "PhoenixMotorControlDevRef"=w326) -> ("error out"=w316:errorcluster, "PhoenixMotorControlDevRef"=w317:T32)  [unwired: 7 in]
  n88 = call <vilib>:"CTRE_Phoenix_MotorControl_ConfigSelectedFeedbackSensor_TalonFX.vi"("error in (no error)"=w316, "Talon FX Feedback Device"=w269, "PhoenixMotorControlDevRef"=w317) -> ("error out"=w314:errorcluster, "PhoenixMotorControlDevRef"=w315:T32)  [unwired: 7 in]
  n89 = call <vilib>:"CTRE_Phoenix_MotorControl_SetSelectedSensorPosition.vi"("error in (no error)"=w314, "pidLoopIdx"=w298, "New Sensor Position"=w299, "PhoenixMotorControlDevRef"=w315) -> ("error out"=w324:errorcluster, "PhoenixMotorControlDevRef"=w323:T32)  [unwired: 6 in]
  n90 = call <vilib>:"CTRE_Phoenix_MotorControl_ConfigOpenLoopRamp.vi"("error in (no error)"=w324, "secondsFromNeutralToFull"=w297, "PhoenixMotorControlDevRef"=w323) -> ("error out"=w320:errorcluster, "PhoenixMotorControlDevRef"=w321:T32)  [unwired: 7 in]
  n91 = call <vilib>:"CTRE_Phoenix_MotorControl_ConfigClosedLoopRamp.vi"("error in (no error)"=w320, "secondsFromNeutralToFull"=w297, "PhoenixMotorControlDevRef"=w321) -> ("error out"=w285:errorcluster, "PhoenixMotorControlDevRef"=w286:T32)  [unwired: 7 in]
  n92 = call <vilib>:"CTRE_Phoenix_MotorControl_ConfigVoltageCompensation.vi"("error in (no error)"=w285, "Saturation Voltage"=w280, "PhoenixMotorControlDevRef"=w286) -> ("error out"=w293:errorcluster, "PhoenixMotorControlDevRef"=w294:T32)  [unwired: 7 in]
  n93 = call <vilib>:"CTRE_Phoenix_MotorControl_EnableVoltageCompensation.vi"("error in (no error)"=w293, "Enable Voltage Compensation?"=w279, "PhoenixMotorControlDevRef"=w294) -> ("error out"=w275:errorcluster, "PhoenixMotorControlDevRef"=w276:T32)  [unwired: 7 in]
  n94 = call <vilib>:"CTRE_Phoenix_MotorControl_OverrideLimitSwitchesEnable.vi"("PhoenixMotorControlDevRef"=w276, "Override Limit Switch Enable?"=w270, "error in (no error)"=w275) -> ("PhoenixMotorControlDevRef"=w259:T32, "error out"=w250:errorcluster)  [unwired: 11 in]
  n95 = call <vilib>:"CTRE_Phoenix_MotorControl_ConfigSupplyCurrentLimit.vi"("error in (no error)"=w250, "Supply Current Limit Configuration"=w256, "PhoenixMotorControlDevRef"=w259) -> ("error out"=w263:errorcluster, "PhoenixMotorControlDevRef"=w264:T32)  [unwired: 7 in]
  n96 = call <vilib>:"CTRE_Phoenix_MotorControl_RefNumRegistrySet.vi"("error in (no error)"=w263, "refnum name"="Drive1", "PhoenixMotorControlDevRef"=w264) -> ("error out"=w244:errorcluster)  [unwired: 7 in, 1 out]
  n97 = call <vilib>:"CTRE_Phoenix_TalonFX_Open.vi"("error in"=w244, "Device Number"=u8 4 ("Drive 4L"), "CAN Bus"=w123) -> ("error out"=w13:errorcluster, "PhoenixMotorControlDevRef"=w14:T32)  [unwired: 7 in]
  n98 = call <vilib>:"CTRE_Phoenix_MotorController_ClearStickyFaults.vi"("error in"=w13, "PhoenixMotorControlDevRef"=w14) -> ("error out"=w332:errorcluster, "PhoenixMotorControlDevRef"=w331:T32)  [unwired: 8 in]
  n99 = call <vilib>:"CTRE_Phoenix_MotorControl_SetInverted_TalonFX.vi"("error in (no error)"=w332, "Invert Type"=w246, "PhoenixMotorControlDevRef"=w331) -> ("error out"=w338:errorcluster, "PhoenixMotorControlDevRef"=w339:T32)  [unwired: 7 in]
  n100 = call <vilib>:"CTRE_Phoenix_MotorControl_SetNeutralMode.vi"("error in (no error)"=w338, "Motor Control Neutral Mode"=w300, "PhoenixMotorControlDevRef"=w339) -> ("error out"=w329:errorcluster, "PhoenixMotorControlDevRef"=w330:T32)  [unwired: 7 in]
  n101 = call <vilib>:"CTRE_Phoenix_MotorControl_ConfigSelectedFeedbackSensor_TalonFX.vi"("error in (no error)"=w329, "Talon FX Feedback Device"=w269, "PhoenixMotorControlDevRef"=w330) -> ("error out"=w327:errorcluster, "PhoenixMotorControlDevRef"=w328:T32)  [unwired: 7 in]
  n102 = call <vilib>:"CTRE_Phoenix_MotorControl_SetSelectedSensorPosition.vi"("error in (no error)"=w327, "pidLoopIdx"=w298, "New Sensor Position"=w299, "PhoenixMotorControlDevRef"=w328) -> ("error out"=w337:errorcluster, "PhoenixMotorControlDevRef"=w336:T32)  [unwired: 6 in]
  n103 = call <vilib>:"CTRE_Phoenix_MotorControl_ConfigOpenLoopRamp.vi"("error in (no error)"=w337, "secondsFromNeutralToFull"=w297, "PhoenixMotorControlDevRef"=w336) -> ("error out"=w333:errorcluster, "PhoenixMotorControlDevRef"=w334:T32)  [unwired: 7 in]
  n104 = call <vilib>:"CTRE_Phoenix_MotorControl_ConfigClosedLoopRamp.vi"("error in (no error)"=w333, "secondsFromNeutralToFull"=w297, "PhoenixMotorControlDevRef"=w334) -> ("error out"=w283:errorcluster, "PhoenixMotorControlDevRef"=w284:T32)  [unwired: 7 in]
  n105 = call <vilib>:"CTRE_Phoenix_MotorControl_ConfigVoltageCompensation.vi"("error in (no error)"=w283, "Saturation Voltage"=w280, "PhoenixMotorControlDevRef"=w284) -> ("error out"=w291:errorcluster, "PhoenixMotorControlDevRef"=w292:T32)  [unwired: 7 in]
  n106 = call <vilib>:"CTRE_Phoenix_MotorControl_EnableVoltageCompensation.vi"("error in (no error)"=w291, "Enable Voltage Compensation?"=w279, "PhoenixMotorControlDevRef"=w292) -> ("error out"=w273:errorcluster, "PhoenixMotorControlDevRef"=w274:T32)  [unwired: 7 in]
  n107 = call <vilib>:"CTRE_Phoenix_MotorControl_OverrideLimitSwitchesEnable.vi"("PhoenixMotorControlDevRef"=w274, "Override Limit Switch Enable?"=w270, "error in (no error)"=w273) -> ("PhoenixMotorControlDevRef"=w258:T32, "error out"=w249:errorcluster)  [unwired: 11 in]
  n108 = call <vilib>:"CTRE_Phoenix_MotorControl_ConfigSupplyCurrentLimit.vi"("error in (no error)"=w249, "Supply Current Limit Configuration"=w256, "PhoenixMotorControlDevRef"=w258) -> ("error out"=w265:errorcluster, "PhoenixMotorControlDevRef"=w266:T32)  [unwired: 7 in]
  n109 = call <vilib>:"CTRE_Phoenix_MotorControl_RefNumRegistrySet.vi"("error in (no error)"=w265, "refnum name"="Drive2", "PhoenixMotorControlDevRef"=w266) -> ("error out"=w243:errorcluster)  [unwired: 7 in, 1 out]
  n110 = call <vilib>:"CTRE_Phoenix_TalonFX_Open.vi"("error in"=w243, "Device Number"=u8 6 ("Drive 4L"), "CAN Bus"=w123) -> ("error out"=w15:errorcluster, "PhoenixMotorControlDevRef"=w16:T32)  [unwired: 7 in]
  n111 = call <vilib>:"CTRE_Phoenix_MotorController_ClearStickyFaults.vi"("error in"=w15, "PhoenixMotorControlDevRef"=w16) -> ("error out"=w345:errorcluster, "PhoenixMotorControlDevRef"=w344:T32)  [unwired: 8 in]
  n112 = call <vilib>:"CTRE_Phoenix_MotorControl_SetInverted_TalonFX.vi"("error in (no error)"=w345, "Invert Type"=w247, "PhoenixMotorControlDevRef"=w344) -> ("error out"=w351:errorcluster, "PhoenixMotorControlDevRef"=w352:T32)  [unwired: 7 in]
  n113 = call <vilib>:"CTRE_Phoenix_MotorControl_SetNeutralMode.vi"("error in (no error)"=w351, "Motor Control Neutral Mode"=w300, "PhoenixMotorControlDevRef"=w352) -> ("error out"=w342:errorcluster, "PhoenixMotorControlDevRef"=w343:T32)  [unwired: 7 in]
  n114 = call <vilib>:"CTRE_Phoenix_MotorControl_ConfigSelectedFeedbackSensor_TalonFX.vi"("error in (no error)"=w342, "Talon FX Feedback Device"=w269, "PhoenixMotorControlDevRef"=w343) -> ("error out"=w340:errorcluster, "PhoenixMotorControlDevRef"=w341:T32)  [unwired: 7 in]
  n115 = call <vilib>:"CTRE_Phoenix_MotorControl_SetSelectedSensorPosition.vi"("error in (no error)"=w340, "pidLoopIdx"=w298, "New Sensor Position"=w299, "PhoenixMotorControlDevRef"=w341) -> ("error out"=w350:errorcluster, "PhoenixMotorControlDevRef"=w349:T32)  [unwired: 6 in]
  n116 = call <vilib>:"CTRE_Phoenix_MotorControl_ConfigOpenLoopRamp.vi"("error in (no error)"=w350, "secondsFromNeutralToFull"=w297, "PhoenixMotorControlDevRef"=w349) -> ("error out"=w346:errorcluster, "PhoenixMotorControlDevRef"=w347:T32)  [unwired: 7 in]
  n117 = call <vilib>:"CTRE_Phoenix_MotorControl_ConfigClosedLoopRamp.vi"("error in (no error)"=w346, "secondsFromNeutralToFull"=w297, "PhoenixMotorControlDevRef"=w347) -> ("error out"=w281:errorcluster, "PhoenixMotorControlDevRef"=w282:T32)  [unwired: 7 in]
  n118 = call <vilib>:"CTRE_Phoenix_MotorControl_ConfigVoltageCompensation.vi"("error in (no error)"=w281, "Saturation Voltage"=w280, "PhoenixMotorControlDevRef"=w282) -> ("error out"=w289:errorcluster, "PhoenixMotorControlDevRef"=w290:T32)  [unwired: 7 in]
  n119 = call <vilib>:"CTRE_Phoenix_MotorControl_EnableVoltageCompensation.vi"("error in (no error)"=w289, "Enable Voltage Compensation?"=w279, "PhoenixMotorControlDevRef"=w290) -> ("error out"=w271:errorcluster, "PhoenixMotorControlDevRef"=w272:T32)  [unwired: 7 in]
  n120 = call <vilib>:"CTRE_Phoenix_MotorControl_OverrideLimitSwitchesEnable.vi"("PhoenixMotorControlDevRef"=w272, "Override Limit Switch Enable?"=w270, "error in (no error)"=w271) -> ("PhoenixMotorControlDevRef"=w257:T32, "error out"=w248:errorcluster)  [unwired: 11 in]
  n121 = call <vilib>:"CTRE_Phoenix_MotorControl_ConfigSupplyCurrentLimit.vi"("error in (no error)"=w248, "Supply Current Limit Configuration"=w256, "PhoenixMotorControlDevRef"=w257) -> ("error out"=w267:errorcluster, "PhoenixMotorControlDevRef"=w268:T32)  [unwired: 7 in]
  n122 = call <vilib>:"CTRE_Phoenix_MotorControl_RefNumRegistrySet.vi"("error in (no error)"=w267, "refnum name"="Drive3", "PhoenixMotorControlDevRef"=w268) -> ("error out"=w158:errorcluster)  [unwired: 7 in, 1 out]
  n123 = call <vilib>:"CTRE_Phoenix_TalonFX_Open.vi"("error in"=w158, "Device Number"=u8 1 ("Drive 4L"), "CAN Bus"=w123) -> ("error out"=w17:errorcluster, "PhoenixMotorControlDevRef"=w18:T32)  [unwired: 7 in]
  n124 = call <vilib>:"CTRE_Phoenix_MotorController_ClearStickyFaults.vi"("error in"=w17, "PhoenixMotorControlDevRef"=w18) -> ("error out"=w217:errorcluster, "PhoenixMotorControlDevRef"=w216:T32)  [unwired: 8 in]
  n125 = call <vilib>:"CTRE_Phoenix_MotorControl_SetInverted_TalonFX.vi"("error in (no error)"=w217, "Invert Type"=w159, "PhoenixMotorControlDevRef"=w216) -> ("error out"=w219:errorcluster, "PhoenixMotorControlDevRef"=w220:T32)  [unwired: 7 in]
  n126 = call <vilib>:"CTRE_Phoenix_MotorControl_SetNeutralMode.vi"("error in (no error)"=w219, "Motor Control Neutral Mode"=w213, "PhoenixMotorControlDevRef"=w220) -> ("error out"=w214:errorcluster, "PhoenixMotorControlDevRef"=w215:T32)  [unwired: 7 in]
  n127 = call <vilib>:"CTRE_Phoenix_MotorControl_ConfigSelectedFeedbackSensor_TalonFX.vi"("error in (no error)"=w214, "Talon FX Feedback Device"=w193, "PhoenixMotorControlDevRef"=w215) -> ("error out"=w166:errorcluster, "PhoenixMotorControlDevRef"=w167:T32)  [unwired: 7 in]
  n128 = call <vilib>:"CTRE_Phoenix_MotorControl_ConfigOpenLoopRamp.vi"("error in (no error)"=w166, "secondsFromNeutralToFull"=w212, "PhoenixMotorControlDevRef"=w167) -> ("PhoenixMotorControlDevRef"=w171:T32)  [unwired: 7 in, 1 out]
  n129 = call <vilib>:"CTRE_Phoenix_MotorControl_ConfigClosedLoopRamp.vi"("secondsFromNeutralToFull"=w212, "PhoenixMotorControlDevRef"=w171) -> ("error out"=w202:errorcluster, "PhoenixMotorControlDevRef"=w203:T32)  [unwired: 8 in]
  n130 = call <vilib>:"CTRE_Phoenix_MotorControl_ConfigVoltageCompensation.vi"("error in (no error)"=w202, "Saturation Voltage"=w195, "PhoenixMotorControlDevRef"=w203) -> ("error out"=w210:errorcluster, "PhoenixMotorControlDevRef"=w211:T32)  [unwired: 7 in]
  n131 = call <vilib>:"CTRE_Phoenix_MotorControl_EnableVoltageCompensation.vi"("error in (no error)"=w210, "Enable Voltage Compensation?"=w194, "PhoenixMotorControlDevRef"=w211) -> ("error out"=w175:errorcluster, "PhoenixMotorControlDevRef"=w184:T32)  [unwired: 7 in]
  n132 = call <vilib>:"CTRE_Phoenix_MotorControl_ConfigSupplyCurrentLimit.vi"("error in (no error)"=w175, "Supply Current Limit Configuration"=w180, "PhoenixMotorControlDevRef"=w184) -> ("error out"=w185:errorcluster, "PhoenixMotorControlDevRef"=w186:T32)  [unwired: 7 in]
  n133 = call <vilib>:"CTRE_Phoenix_MotorControl_RefNumRegistrySet.vi"("error in (no error)"=w185, "refnum name"="Turn0", "PhoenixMotorControlDevRef"=w186) -> ("error out"=w48:errorcluster)  [unwired: 7 in, 1 out]
  n134 = call <vilib>:"CTRE_Phoenix_TalonFX_Open.vi"("error in"=w48, "Device Number"=u8 3 ("Drive 4L"), "CAN Bus"=w123) -> ("error out"=w19:errorcluster, "PhoenixMotorControlDevRef"=w20:T32)  [unwired: 7 in]
  n135 = call <vilib>:"CTRE_Phoenix_MotorController_ClearStickyFaults.vi"("error in"=w19, "PhoenixMotorControlDevRef"=w20) -> ("error out"=w224:errorcluster, "PhoenixMotorControlDevRef"=w223:T32)  [unwired: 8 in]
  n136 = call <vilib>:"CTRE_Phoenix_MotorControl_SetInverted_TalonFX.vi"("error in (no error)"=w224, "Invert Type"=w159, "PhoenixMotorControlDevRef"=w223) -> ("error out"=w226:errorcluster, "PhoenixMotorControlDevRef"=w227:T32)  [unwired: 7 in]
  n137 = call <vilib>:"CTRE_Phoenix_MotorControl_SetNeutralMode.vi"("error in (no error)"=w226, "Motor Control Neutral Mode"=w213, "PhoenixMotorControlDevRef"=w227) -> ("error out"=w221:errorcluster, "PhoenixMotorControlDevRef"=w222:T32)  [unwired: 7 in]
  n138 = call <vilib>:"CTRE_Phoenix_MotorControl_ConfigSelectedFeedbackSensor_TalonFX.vi"("error in (no error)"=w221, "Talon FX Feedback Device"=w193, "PhoenixMotorControlDevRef"=w222) -> ("error out"=w164:errorcluster, "PhoenixMotorControlDevRef"=w165:T32)  [unwired: 7 in]
  n139 = call <vilib>:"CTRE_Phoenix_MotorControl_ConfigOpenLoopRamp.vi"("error in (no error)"=w164, "secondsFromNeutralToFull"=w212, "PhoenixMotorControlDevRef"=w165) -> ("PhoenixMotorControlDevRef"=w170:T32)  [unwired: 7 in, 1 out]
  n140 = call <vilib>:"CTRE_Phoenix_MotorControl_ConfigClosedLoopRamp.vi"("secondsFromNeutralToFull"=w212, "PhoenixMotorControlDevRef"=w170) -> ("error out"=w200:errorcluster, "PhoenixMotorControlDevRef"=w201:T32)  [unwired: 8 in]
  n141 = call <vilib>:"CTRE_Phoenix_MotorControl_ConfigVoltageCompensation.vi"("error in (no error)"=w200, "Saturation Voltage"=w195, "PhoenixMotorControlDevRef"=w201) -> ("error out"=w208:errorcluster, "PhoenixMotorControlDevRef"=w209:T32)  [unwired: 7 in]
  n142 = call <vilib>:"CTRE_Phoenix_MotorControl_EnableVoltageCompensation.vi"("error in (no error)"=w208, "Enable Voltage Compensation?"=w194, "PhoenixMotorControlDevRef"=w209) -> ("error out"=w174:errorcluster, "PhoenixMotorControlDevRef"=w183:T32)  [unwired: 7 in]
  n143 = call <vilib>:"CTRE_Phoenix_MotorControl_ConfigSupplyCurrentLimit.vi"("error in (no error)"=w174, "Supply Current Limit Configuration"=w180, "PhoenixMotorControlDevRef"=w183) -> ("error out"=w187:errorcluster, "PhoenixMotorControlDevRef"=w188:T32)  [unwired: 7 in]
  n144 = call <vilib>:"CTRE_Phoenix_MotorControl_RefNumRegistrySet.vi"("error in (no error)"=w187, "refnum name"="Turn1", "PhoenixMotorControlDevRef"=w188) -> ("error out"=w47:errorcluster)  [unwired: 7 in, 1 out]
  n145 = call <vilib>:"CTRE_Phoenix_TalonFX_Open.vi"("error in"=w47, "Device Number"=u8 5 ("Drive 4L"), "CAN Bus"=w123) -> ("error out"=w21:errorcluster, "PhoenixMotorControlDevRef"=w22:T32)  [unwired: 7 in]
  n146 = call <vilib>:"CTRE_Phoenix_MotorController_ClearStickyFaults.vi"("error in"=w21, "PhoenixMotorControlDevRef"=w22) -> ("error out"=w231:errorcluster, "PhoenixMotorControlDevRef"=w230:T32)  [unwired: 8 in]
  n147 = call <vilib>:"CTRE_Phoenix_MotorControl_SetInverted_TalonFX.vi"("error in (no error)"=w231, "Invert Type"=w159, "PhoenixMotorControlDevRef"=w230) -> ("error out"=w233:errorcluster, "PhoenixMotorControlDevRef"=w234:T32)  [unwired: 7 in]
  n148 = call <vilib>:"CTRE_Phoenix_MotorControl_SetNeutralMode.vi"("error in (no error)"=w233, "Motor Control Neutral Mode"=w213, "PhoenixMotorControlDevRef"=w234) -> ("error out"=w228:errorcluster, "PhoenixMotorControlDevRef"=w229:T32)  [unwired: 7 in]
  n149 = call <vilib>:"CTRE_Phoenix_MotorControl_ConfigSelectedFeedbackSensor_TalonFX.vi"("error in (no error)"=w228, "Talon FX Feedback Device"=w193, "PhoenixMotorControlDevRef"=w229) -> ("error out"=w162:errorcluster, "PhoenixMotorControlDevRef"=w163:T32)  [unwired: 7 in]
  n150 = call <vilib>:"CTRE_Phoenix_MotorControl_ConfigOpenLoopRamp.vi"("error in (no error)"=w162, "secondsFromNeutralToFull"=w212, "PhoenixMotorControlDevRef"=w163) -> ("PhoenixMotorControlDevRef"=w169:T32)  [unwired: 7 in, 1 out]
  n151 = call <vilib>:"CTRE_Phoenix_MotorControl_ConfigClosedLoopRamp.vi"("secondsFromNeutralToFull"=w212, "PhoenixMotorControlDevRef"=w169) -> ("error out"=w198:errorcluster, "PhoenixMotorControlDevRef"=w199:T32)  [unwired: 8 in]
  n152 = call <vilib>:"CTRE_Phoenix_MotorControl_ConfigVoltageCompensation.vi"("error in (no error)"=w198, "Saturation Voltage"=w195, "PhoenixMotorControlDevRef"=w199) -> ("error out"=w206:errorcluster, "PhoenixMotorControlDevRef"=w207:T32)  [unwired: 7 in]
  n153 = call <vilib>:"CTRE_Phoenix_MotorControl_EnableVoltageCompensation.vi"("error in (no error)"=w206, "Enable Voltage Compensation?"=w194, "PhoenixMotorControlDevRef"=w207) -> ("error out"=w173:errorcluster, "PhoenixMotorControlDevRef"=w182:T32)  [unwired: 7 in]
  n154 = call <vilib>:"CTRE_Phoenix_MotorControl_ConfigSupplyCurrentLimit.vi"("error in (no error)"=w173, "Supply Current Limit Configuration"=w180, "PhoenixMotorControlDevRef"=w182) -> ("error out"=w189:errorcluster, "PhoenixMotorControlDevRef"=w190:T32)  [unwired: 7 in]
  n155 = call <vilib>:"CTRE_Phoenix_MotorControl_RefNumRegistrySet.vi"("error in (no error)"=w189, "refnum name"="Turn2", "PhoenixMotorControlDevRef"=w190) -> ("error out"=w46:errorcluster)  [unwired: 7 in, 1 out]
  n156 = call <vilib>:"CTRE_Phoenix_TalonFX_Open.vi"("error in"=w46, "Device Number"=u8 7 ("Drive 4L"), "CAN Bus"=w123) -> ("error out"=w23:errorcluster, "PhoenixMotorControlDevRef"=w24:T32)  [unwired: 7 in]
  n157 = call <vilib>:"CTRE_Phoenix_MotorController_ClearStickyFaults.vi"("error in"=w23, "PhoenixMotorControlDevRef"=w24) -> ("error out"=w238:errorcluster, "PhoenixMotorControlDevRef"=w237:T32)  [unwired: 8 in]
  n158 = call <vilib>:"CTRE_Phoenix_MotorControl_SetInverted_TalonFX.vi"("error in (no error)"=w238, "Invert Type"=w159, "PhoenixMotorControlDevRef"=w237) -> ("error out"=w240:errorcluster, "PhoenixMotorControlDevRef"=w241:T32)  [unwired: 7 in]
  n159 = call <vilib>:"CTRE_Phoenix_MotorControl_SetNeutralMode.vi"("error in (no error)"=w240, "Motor Control Neutral Mode"=w213, "PhoenixMotorControlDevRef"=w241) -> ("error out"=w235:errorcluster, "PhoenixMotorControlDevRef"=w236:T32)  [unwired: 7 in]
  n160 = call <vilib>:"CTRE_Phoenix_MotorControl_ConfigSelectedFeedbackSensor_TalonFX.vi"("error in (no error)"=w235, "Talon FX Feedback Device"=w193, "PhoenixMotorControlDevRef"=w236) -> ("error out"=w160:errorcluster, "PhoenixMotorControlDevRef"=w161:T32)  [unwired: 7 in]
  n161 = call <vilib>:"CTRE_Phoenix_MotorControl_ConfigOpenLoopRamp.vi"("error in (no error)"=w160, "secondsFromNeutralToFull"=w212, "PhoenixMotorControlDevRef"=w161) -> ("PhoenixMotorControlDevRef"=w168:T32)  [unwired: 7 in, 1 out]
  n162 = call <vilib>:"CTRE_Phoenix_MotorControl_ConfigClosedLoopRamp.vi"("secondsFromNeutralToFull"=w212, "PhoenixMotorControlDevRef"=w168) -> ("error out"=w196:errorcluster, "PhoenixMotorControlDevRef"=w197:T32)  [unwired: 8 in]
  n163 = call <vilib>:"CTRE_Phoenix_MotorControl_ConfigVoltageCompensation.vi"("error in (no error)"=w196, "Saturation Voltage"=w195, "PhoenixMotorControlDevRef"=w197) -> ("error out"=w204:errorcluster, "PhoenixMotorControlDevRef"=w205:T32)  [unwired: 7 in]
  n164 = call <vilib>:"CTRE_Phoenix_MotorControl_EnableVoltageCompensation.vi"("error in (no error)"=w204, "Enable Voltage Compensation?"=w194, "PhoenixMotorControlDevRef"=w205) -> ("error out"=w172:errorcluster, "PhoenixMotorControlDevRef"=w181:T32)  [unwired: 7 in]
  n165 = call <vilib>:"CTRE_Phoenix_MotorControl_ConfigSupplyCurrentLimit.vi"("error in (no error)"=w172, "Supply Current Limit Configuration"=w180, "PhoenixMotorControlDevRef"=w181) -> ("error out"=w191:errorcluster, "PhoenixMotorControlDevRef"=w192:T32)  [unwired: 7 in]
  n166 = call <vilib>:"CTRE_Phoenix_MotorControl_RefNumRegistrySet.vi"("error in (no error)"=w191, "refnum name"="Turn3", "PhoenixMotorControlDevRef"=w192) -> ()  [unwired: 7 in, 2 out]
  n167 = call <vilib>:"Spark MAX Set Inverted.vi"("error in (no error)"=w127, "Inverted (F)"=FALSE, "MotorControlDeviceRef in"=w126) -> ("error out"=w105:errorcluster, "MotorControlDeviceRef out"=w104:T32)  [unwired: 7 in]
  n168 = call <vilib>:"Spark MAX Set Soft Limit Config.vi"("error in (no error)"=w105, "Soft Limit (0)"=-0.1, "Soft Limit Switch"=Spark_MAX_Limit_Direction."Forward Limit", "MotorControlDeviceRef in"=w104) -> ("error out"=w101:errorcluster, "MotorControlDeviceRef out"=w102:T32)  [unwired: 6 in]
  n169 = call <vilib>:"Spark MAX Set Soft Limit Config.vi"("error in (no error)"=w101, "Soft Limit (0)"=-85.0, "Soft Limit Switch"=Spark_MAX_Limit_Direction."Reverse Limit", "MotorControlDeviceRef in"=w102) -> ("error out"=w100:errorcluster, "MotorControlDeviceRef out"=w99:T32)  [unwired: 6 in]
  n170 = call <vilib>:"WPI_MotorControlRefNum Registry Set.vi"("error in (no error)"=w100, "refnum name"="Escalator", "MotorControlDevRef"=w99) -> ("error out"=w115:errorcluster)  [unwired: 7 in, 1 out]
  n171 = call <vilib>:"Spark MAX Open.vi"("error in (no error)"=w115, "Device Number"=u8 2) -> ("error out"=w39:errorcluster, "MotorControlDeviceRef"=w38:T32)  [unwired: 8 in]
  n172 = call <vilib>:"Spark MAX Set Smart Current Limit.vi"("error in (no error)"=w39, "Free Speed Current Limit (20A)"=w42, "Primay Current Limit (80A)"=w43, "MotorControlDeviceRef in"=w38) -> ("error out"=w51:errorcluster, "MotorControlDeviceRef out"=w52:T32)  [unwired: 6 in]
  n173 = call <vilib>:"Spark MAX Set Idle Mode.vi"("error in (no error)"=w51, "MotorControlDeviceRef in"=w52) -> ("error out"=w120:errorcluster, "MotorControlDeviceRef out"=w121:T32)  [unwired: 8 in]
  n174 = call <vilib>:"Spark MAX Set Inverted.vi"("error in (no error)"=w120, "Inverted (F)"=FALSE, "MotorControlDeviceRef in"=w121) -> ("error out"=w119:errorcluster, "MotorControlDeviceRef out"=w118:T32)  [unwired: 7 in]
  n175 = call <vilib>:"WPI_MotorControlRefNum Registry Set.vi"("error in (no error)"=w119, "refnum name"="In.Bot", "MotorControlDevRef"=w118) -> ("error out"=w107:errorcluster)  [unwired: 7 in, 1 out]
  n176 = call <vilib>:"Spark MAX Open.vi"("error in (no error)"=w107, "Device Number"=u8 3) -> ("error out"=w41:errorcluster, "MotorControlDeviceRef"=w40:T32)  [unwired: 8 in]
  n177 = call <vilib>:"Spark MAX Set Smart Current Limit.vi"("error in (no error)"=w41, "Free Speed Current Limit (20A)"=w42, "Primay Current Limit (80A)"=w43, "MotorControlDeviceRef in"=w40) -> ("error out"=w50:errorcluster, "MotorControlDeviceRef out"=w49:T32)  [unwired: 6 in]
  n178 = call <vilib>:"Spark MAX Set Idle Mode.vi"("error in (no error)"=w50, "Idle Mode"=Spark_MAX_Idle_Mode."Coast", "MotorControlDeviceRef in"=w49) -> ("error out"=w112:errorcluster, "MotorControlDeviceRef out"=w111:T32)  [unwired: 7 in]
  n179 = call <vilib>:"Spark MAX Set Inverted.vi"("error in (no error)"=w112, "Inverted (F)"=FALSE, "MotorControlDeviceRef in"=w111) -> ("error out"=w113:errorcluster, "MotorControlDeviceRef out"=w114:T32)  [unwired: 7 in]
  n180 = call <vilib>:"WPI_MotorControlRefNum Registry Set.vi"("error in (no error)"=w113, "refnum name"="In.Top", "MotorControlDevRef"=w114) -> ("error out"=w34:errorcluster)  [unwired: 7 in, 1 out]
  n181 = call-poly <vilib>:"WPI_MotorControlOpen.vi"("error in (no error)"=w34, "PWM Channel"=FPGA_DIOPWMChannel."PWM 9") -> ("error out"=w33:errorcluster, "MotorControlDeviceRef"=w32:T32)  [unwired: 8 in]
  n182 = call <vilib>:"WPI_MotorControlRefNum Registry Set.vi"("error in (no error)"=w33, "refnum name"="LEDS", "MotorControlDevRef"=w32) -> ()  [unwired: 7 in, 2 out]
  "error out" <- "error in"
